vi "Core Cleanup.vi"(8 "error in (no error)":errorcluster, 11 "CIFTemplateNode in":refnum<class "CIFCorePlugin.lvclass">) -> (0 "error out":errorcluster, 3 "CIFTemplateNode out":refnum<class "CIFCorePlugin.lvclass">)   [LabVIEW 2021, in "CIFCorePlugin.lvclass"]
uses:
  CIFCorePlugin.lvclass
  CIFCorePlugin.lvclass/CIFCorePlugin.ctl
  CIFCoreCommon/Typedef/Plugin State.ctl
  Typedef/Energized States.ctl
  CIFUtilities/CIFClocks/Core/Get Time.vi
  CIFCoreCommon/Utilities/Update Delta Time.vi
  Accessors/Timestamps/Read Cleanup TS.vi
  Accessors/Get Time.vi
  CIFUtilities/CIFClocks/Time Conversion/LabVIEW Time to UTC Time.vi
  CIFUtilities/CIFClocks/SubVIs/Add Error.vi
  CIFCoreCommon/CIFCoreCommon.lvlib
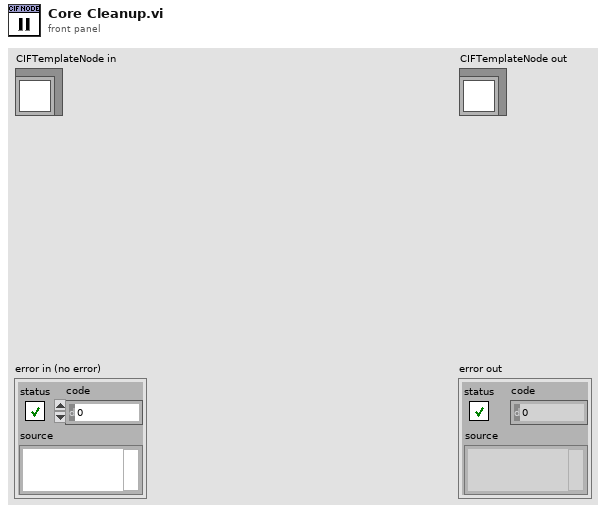
[diagram p1: front panel]
types:
  T1 = typedef "CIFCorePlugin.lvclass/Energized States.ctl" = enum16{"Listen", "Prepare", "Execute", "Housekeep", "Cleanup", "Destroy"}
  T2 = typedef "CIFCoreCommon.lvlib/Plugin State.ctl" = enum32{"Null", "Creating", "Listening", "Running", "CleaningUp", "Destroying"}
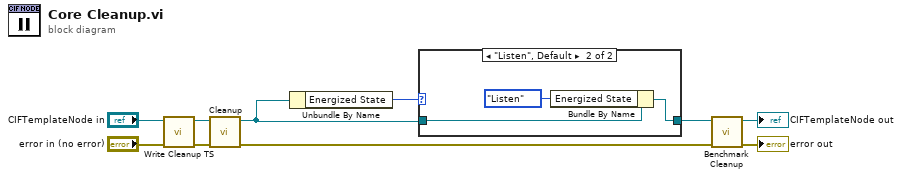
[diagram p0: block diagram]
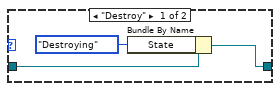
[diagram p2: hidden frame]
diagram:
  n1 = call "Write Cleanup TS.vi"("error in (no error)"="error in (no error)", "CIFCorePlugin in"="CIFTemplateNode in") -> ("error out"=w3:errorcluster, "CIFCorePlugin out"=w2:refnum<class "CIFCorePlugin.lvclass">)  [unwired: 8 in]
  n2 = call-dynamic "Cleanup.vi"("error in (no error)"=w3, "CIFTemplateNode in"=w2) -> ("error out"=w7:errorcluster, "CIFTemplateNode out"=w9:refnum<class "CIFCorePlugin.lvclass">)  [unwired: 8 in]
  n3 = Unbundle By Name(w9) -> ("Energized State"=w10:T1)
  n4 = case shown="\"Listen\", Default" w10 {
    tunnel: w9 -> [w12 w16]
    tunnel: [w11 w15] -> w8
    frame "Destroy" {
      n5 = Bundle By Name(cluster=w12, "State"=Plugin_State."Destroying" ("Status.State")) -> (w11:refnum<class "CIFCorePlugin.lvclass">)
    }
    frame "Listen", Default {
      n6 = Bundle By Name(cluster=w16, "Energized State"=Energized_States."Listen") -> (w15:refnum<class "CIFCorePlugin.lvclass">)
    }
  }
  n7 = call "Benchmark Cleanup.vi"("error in (no error)"=w7, "CIFCorePlugin in"=w8) -> ("error out"=→"error out":errorcluster, "CIFCorePlugin out"=→"CIFTemplateNode out":refnum<class "CIFCorePlugin.lvclass">)  [unwired: 8 in]
